vi "task4_BINARY2DEC_CONVERTER_MORE_DISPLAY.vi"() -> ()   [LabVIEW 2017]
panel:
  out "Tank":dbl(slide) scale=0.0..300.0
  out "Meter":dbl(knob) scale=0.0..300.0
  out "Gauge":dbl(knob) scale=0.0..300.0
  out "display":dbl
  in  "2^0":bool
  in  "2^1":bool
  in  "2^2":bool
  in  "2^3":bool
  in  "2^4":bool
  in  "2^5":bool
  in  "2^6":bool
  in  "2^7":bool
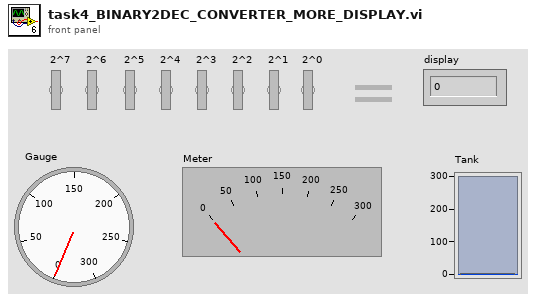
[diagram p1: front panel]
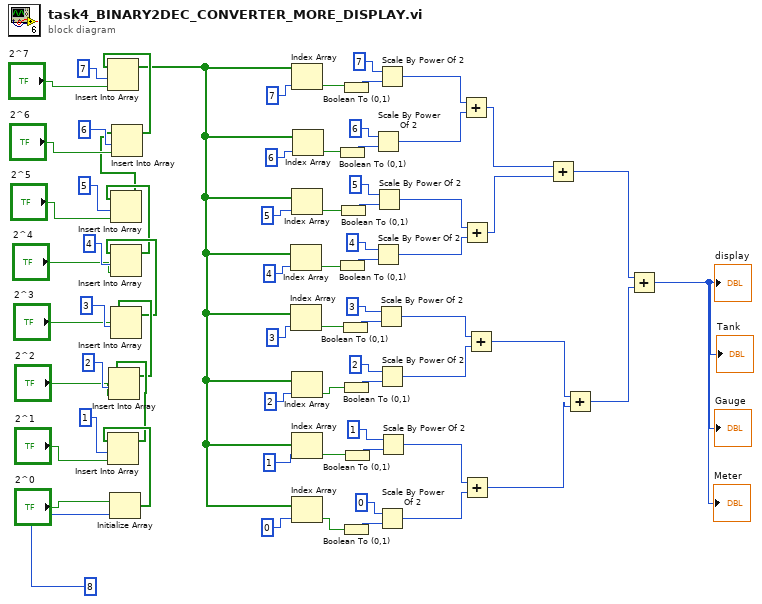
[diagram p0: block diagram]
diagram:
  n1 = Initialize Array("2^0", 8) -> (w8:bool[])
  n2 = Insert Into Array(array=w8, index=1, new element="2^1") -> (w7:bool[])
  n3 = Insert Into Array(array=w7, index=2, new element="2^2") -> (w6:bool[])
  n4 = Insert Into Array(array=w6, index=3, new element="2^3") -> (w5:bool[])
  n5 = Insert Into Array(array=w5, index=4, new element="2^4") -> (w4:bool[])
  n6 = Insert Into Array(array=w4, index=5, new element="2^5") -> (w3:bool[])
  n7 = Insert Into Array(array=w3, index=6, new element="2^6") -> (w2:bool[])
  n8 = Insert Into Array(array=w2, index=7, new element="2^7") -> (w1:bool[])
  n9 = Index Array(array=w1, index=4) -> (element=w16:bool)
  n10 = Index Array(array=w1, index=3) -> (element=w27:bool)
  n11 = Index Array(array=w1, index=7) -> (element=w19:bool)
  n12 = Index Array(array=w1, index=5) -> (element=w17:bool)
  n13 = Index Array(array=w1, index=2) -> (element=w15:bool)
  n14 = Index Array(array=w1, index=1) -> (element=w14:bool)
  n15 = Index Array(array=w1, index=0) -> (element=w13:bool)
  n16 = Index Array(array=w1, index=6) -> (element=w18:bool)
  n17 = Boolean To (0,1)(Boolean=w18) -> (0, 1=w65:i16)
  n18 = Boolean To (0,1)(Boolean=w16) -> (0, 1=w67:i16)
  n19 = Boolean To (0,1)(Boolean=w17) -> (0, 1=w66:i16)
  n20 = Boolean To (0,1)(Boolean=w27) -> (0, 1=w68:i16)
  n21 = Boolean To (0,1)(Boolean=w19) -> (0, 1=w64:i16)
  n22 = Boolean To (0,1)(Boolean=w15) -> (0, 1=w69:i16)
  n23 = Boolean To (0,1)(Boolean=w13) -> (0, 1=w71:i16)
  n24 = Boolean To (0,1)(Boolean=w14) -> (0, 1=w70:i16)
  n25 = Scale By Power Of 2(n=6, x=w65) -> (x*2^n=w54:i16)
  n26 = Scale By Power Of 2(n=4, x=w67) -> (x*2^n=w52:i16)
  n27 = Scale By Power Of 2(n=5, x=w66) -> (x*2^n=w53:i16)
  n28 = Scale By Power Of 2(n=3, x=w68) -> (x*2^n=w51:i16)
  n29 = Scale By Power Of 2(n=7, x=w64) -> (x*2^n=w55:i16)
  n30 = Scale By Power Of 2(n=2, x=w69) -> (x*2^n=w50:i16)
  n31 = Scale By Power Of 2(n=0, x=w71) -> (x*2^n=w48:i16)
  n32 = Scale By Power Of 2(n=1, x=w70) -> (x*2^n=w49:i16)
  n33 = Add(x=w55, y=w54) -> (x+y=w44:i16)
  n34 = Add(x=w53, y=w52) -> (x+y=w45:i16)
  n35 = Add(x=w49, y=w48) -> (x+y=w46:i16)
  n36 = Add(x=w51, y=w50) -> (x+y=w47:i16)
  n37 = Add(x=w44, y=w45) -> (x+y=w43:i16)
  n38 = Add(x=w47, y=w46) -> (x+y=w42:i16)
  n39 = Add(x=w43, y=w42) -> (x+y=→"display" →"Gauge" →"Meter" →"Tank":i16)
